vi "dot2coma.vi"(9 "Data type":u16(ring), 11 "string from file":string[][](array[string])) -> (2 "units":string[][](array[string]), 3 "force curve":dbl[][](array[numeric]))   [LabVIEW 2015]
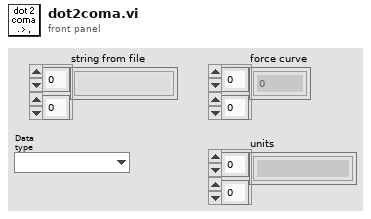
[diagram p1: front panel]
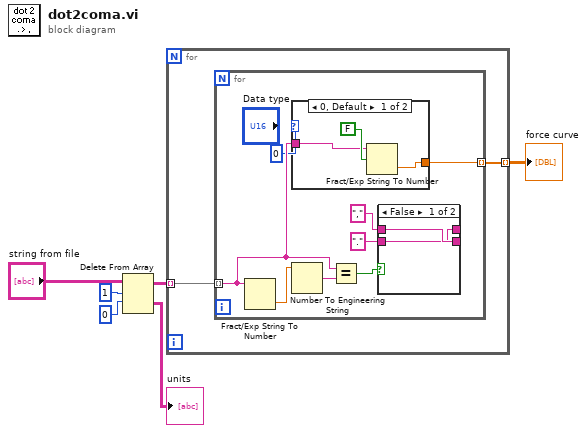
[diagram p0: block diagram]
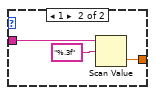
[diagram p2: hidden frame]
diagram:
  n1 = Delete From Array(array="string from file", length=1, index (row)=0) -> (deleted portion=→"units":string[][], array with subset deleted=w4:string[][])  [unwired: 1 in]
  n2 = for {
    tunnel: w4 -> [w8] mode=indexing
    tunnel: [w7] -> w5 mode=indexing
    n3 = for {
      tunnel: w8 -> [w10] mode=indexing
      tunnel: [w16] -> w7 mode=indexing
      n4 = Fract/Exp String To Number(string=w10) -> (number=w14:dbl)  [unwired: 3 in, 1 out]
      n5 = case shown="0, Default" u16 0 ("Ring") {
        tunnel: [w17 w21] -> w16
        tunnel: w10 -> [w18 w20]
        frame 0, Default {
          n6 = Fract/Exp String To Number(use system decimal point (T)=FALSE, string=w18) -> (number=w17:dbl)  [unwired: 2 in, 1 out]
        }
        frame 1 {
          n7 = Scan Value(string=w20, format string="%.3f" ("type")) -> (value=w21:dbl)  [unwired: 1 in, 1 out]
        }
      }
      n8 = Number To Engineering String(4:w14) -> (0:w15:string)  [unwired: 3 in]
      n9 = Equal?(x=w10, y=w15) -> (x = y?=w13:bool)
      n10 = case shown="False" w13 {
        tunnel: [w24 w25] -> _
        tunnel: [w23 w26] -> _
        tunnel: "," -> [w24 w26]
        tunnel: "." -> [w23 w25]
        frame False {
        }
        frame True {
        }
      }
    }
  }
  "force curve" <- w5
